vi "CB Update Controller.vi"(4 "r(k+1)":dbl[](array[numeric]), 6 "Feed Forward":T2, 8 "State Space Model":T1, 9 "x_hat":dbl[](array[numeric]), 10 "r(k)":dbl[](array[numeric]), 11 "K":T2) -> (3 "u":dbl[](array[numeric]))   [LabVIEW 2020]
uses:
  <vilib>/Analysis/Matrix/Datatypes/RealMatrix.ctl
  CB State Space.ctl
  <vilib>/Analysis/baseanly.llb/A x Vector.vi
  <vilib>/Analysis/NI_AALBase.lvlib
  <vilib>/Analysis/Matrix/NI_Matrix.lvlib
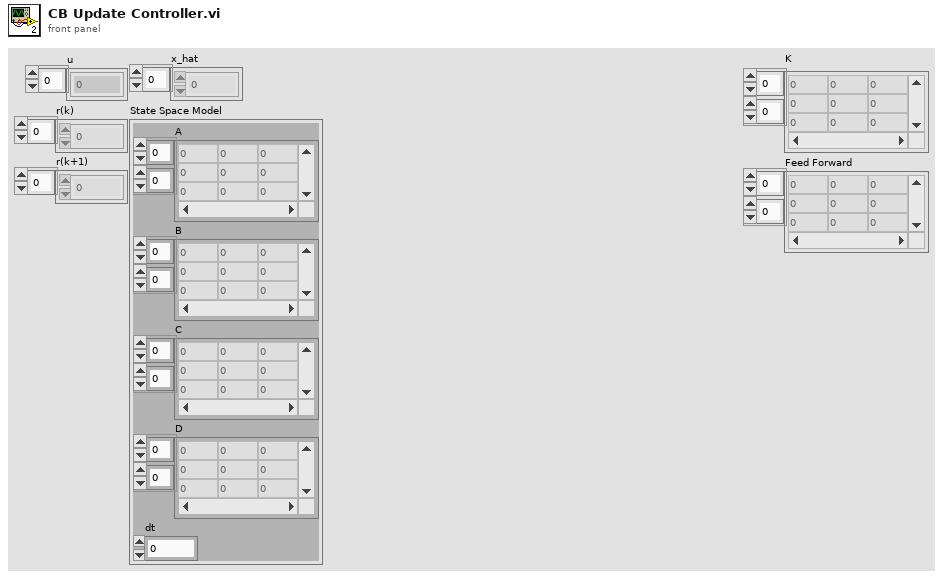
[diagram p1: front panel]
types:
  T1 = typedef "CB State Space.ctl" = cluster{"A":T2, "B":T2, "C":T2, "D":T2, "dt":dbl}
  T2 = typedef "NI_Matrix.lvlib/RealMatrix.ctl" = dbl[][]
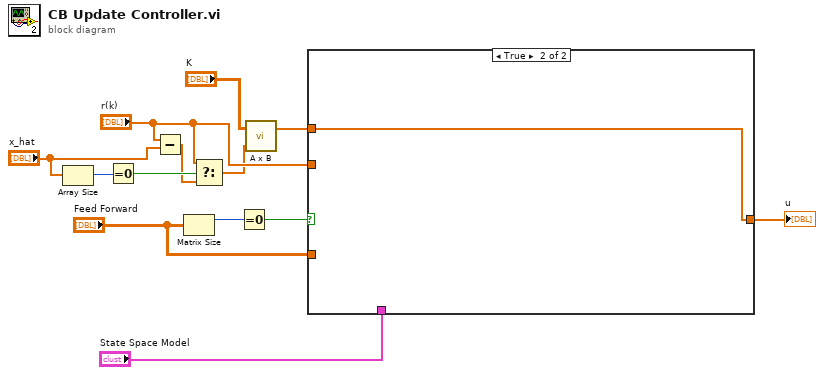
[diagram p0: block diagram]
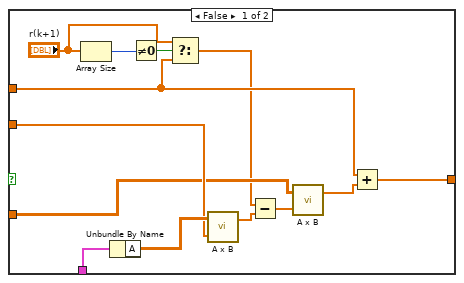
[diagram p2: hidden frame]
diagram:
  n1 = Array Size(array="x_hat") -> (size(s)=w5:i32)
  n2 = Equal To 0?(x=w5) -> (x = 0?=w4:bool)
  n3 = Subtract(x="r(k)", y="x_hat") -> (x-y=w2:dbl[])
  n4 = Matrix Size(0:"Feed Forward") -> (1:w12:i32)  [unwired: 1 out]
  n5 = Select(t="r(k)", s=w4, f=w2) -> (s? t:f=w1:dbl[])
  n6 = Equal To 0?(x=w12) -> (x = 0?=w13:bool)
  n7 = call-poly <vilib>:"A x B.vi"("Vector"=w1, "A"="K") -> ("A x Vector"=w7:dbl[])  [unwired: 1 out]
  n8 = case shown="True" w13 {
    tunnel: w7 -> [w15 w27]
    tunnel: "Feed Forward" -> [w21 _]
    tunnel: "State Space Model" -> [w26 _]
    tunnel: "r(k)" -> [w23 _]
    tunnel: [w19 w27] -> w8
    frame False {
      n9 = Array Size(array="r(k+1)") -> (size(s)=w16:i32)
      n10 = Unbundle By Name(w26) -> ("A"=w25:T2)
      n11 = Not Equal To 0?(x=w16) -> (x != 0?=w17:bool)
      n12 = Select(t="r(k+1)", s=w17, f=w15) -> (s? t:f=w14:dbl[])
      n13 = call-poly <vilib>:"A x B.vi"("Vector"=w23, "A"=w25) -> ("A x Vector"=w24:dbl[])  [unwired: 1 out]
      n14 = Subtract(x=w14, y=w24) -> (x-y=w22:dbl[])
      n15 = call-poly <vilib>:"A x B.vi"("Vector"=w22, "A"=w21) -> ("A x Vector"=w20:dbl[])  [unwired: 1 out]
      n16 = Add(x=w15, y=w20) -> (x+y=w19:dbl[])
    }
    frame True {
    }
  }
  "u" <- w8
